vi "Mood to Image.vi"(11 "Mood":string) -> (3 "Image number":u16)   [LabVIEW 2026]
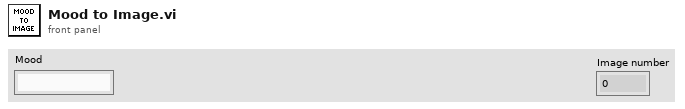
[diagram p1: front panel]
types:
  T1 = enum16{"Happy", "Sad", "Hungry", "Dirty", "Sleepy", "Bug Fixing Happy Dance", "Ate Spaghetti (Code) Until Sick", "Broken Arrow Again?! I'm done!"}
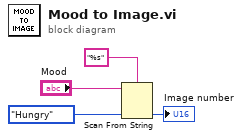
[diagram p0: block diagram]
diagram:
  n1 = Scan From String(format string="%s", input string="Mood", default 1=T1."Hungry") -> (output 1=→"Image number":T1)  [unwired: 2 in, 3 out]
